vi "KeyEvent.vi"() -> ()   [LabVIEW 2019]
panel:
  in  "Ordem de serviço":string
  out "SO code":string
  in  "stop":bool
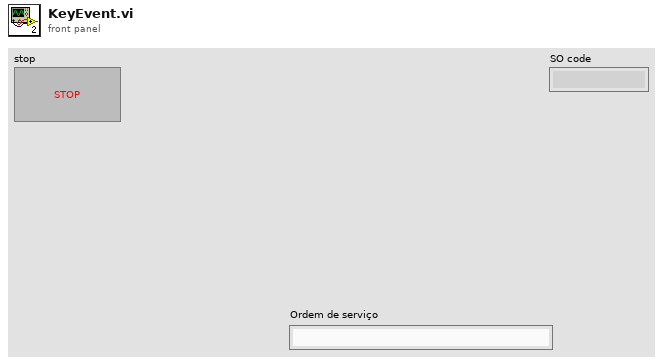
[diagram p1: front panel]
types:
  T1 = cluster{"New data?":bool, "Current QR code":string, "Read code on next":bool}
  T2 = cluster{"New data?":bool, "SO code":string, "Read code on next":bool}
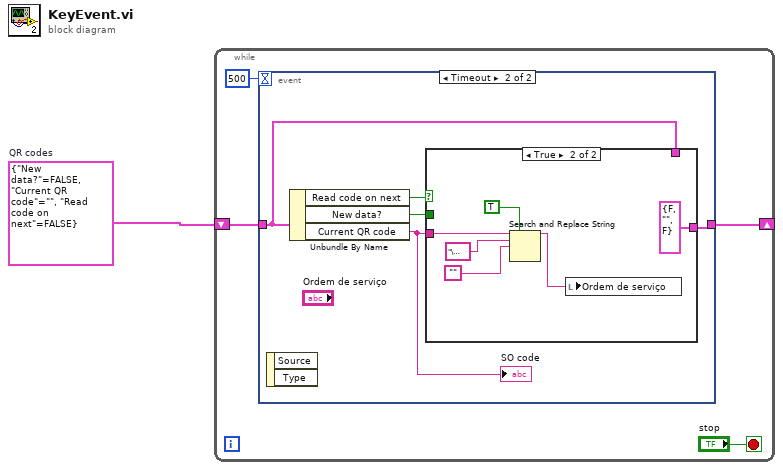
[diagram p0: block diagram]
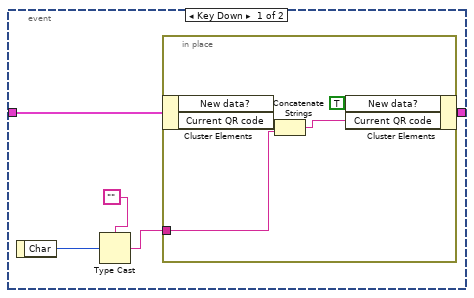
[diagram p2: hidden frame]
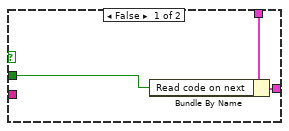
[diagram p3: hidden frame]
diagram:
  w1 = T1 {"New data?"=FALSE, "Current QR code"="", "Read code on next"=FALSE}  # QR codes
  n1 = while {
    shift-right: [w3] -> _
    shift-left: w1 -> [w4]
    stop <- "stop" stop-if-true
    n2 = event shown="[1] Timeout" {
      selector: _ -> [_ _]
      dyn-events: _ -> [_ _]
      timeout: 500 -> [_ _]
      tunnel: w4 -> [w9 w19]
      tunnel: [w7 w18] -> w3
      event Key Down {
        n3 = event-data() -> ("Char"=w10:i16)  [unwired: 1 in]
        n4 = Type Cast(type="", x=w10) -> (*(type *) &x=w8:string)
        n5 = in-place {
          in-place-border: w8 -> [w13]
          n6 = in-place-cluster #1(w9) -> ("Current QR code"=w14:string)  [unwired: 1 out]
          n7 = Concatenate Strings(w14, w13) -> (w12:string)
          n8 = in-place-cluster #1("New data?"=TRUE, "Current QR code"=w12) -> (w7:T1)
        }
      }
      event Timeout {
        n9 = event-data() -> ()  [unwired: 1 in, 2 out]
        n10 = Unbundle By Name(w19) -> ("Read code on next"=w16:bool, "New data?"=w17:bool, "Current QR code"=w15:string)
        "SO code" <- w15
        n11 = case shown="True" w16 {
          tunnel: w19 -> [w22 _]
          tunnel: [w21 T2 {"New data?"=FALSE, "SO code"="", "Read code on next"=FALSE}] -> w18
          tunnel: w17 -> [w20 _]
          tunnel: w15 -> [_ w26]
          frame False {
            n12 = Bundle By Name(cluster=w22, "Read code on next"=w20) -> (w21:T1)
          }
          frame True {
            n13 = Search and Replace String(replace all?=TRUE ("replace all? (F)"), input string=w26, search string="\u0000", replace string="") -> (result string=w25:string)  [unwired: 4 in, 3 out]
            n14 = local write "Ordem de serviço"(w25) -> ()
          }
        }
      }
    }
  }
